vi "WRITE XNET Init Settings.vi"(7 "Unit Type":T1, 8 "error in (no error)":errorcluster, 9 "Box IDs":u8[](array[numeric])=[1], 10 "CAN Interface":refnum<k21>, 11 "XNET_BS120x in":refnum<class "XNET_BS120x.lvclass">) -> (0 "error out":errorcluster, 3 "XNET_BS120x out":refnum<class "XNET_BS120x.lvclass">)   [LabVIEW 2021, in "BS120x Driver.lvlib" / "XNET_BS120x.lvclass"]
uses:
  XNET_BS120x.lvclass
  XNET_BS120x.lvclass/XNET_BS120x.ctl
  TypeDefs/UnitType.ctl
  BS120x.lvclass
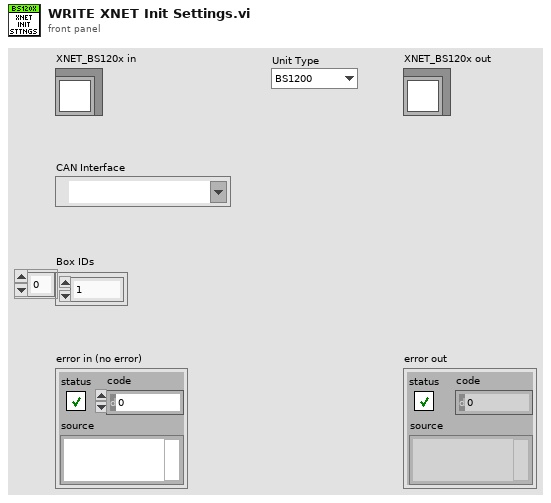
[diagram p1: front panel]
types:
  T1 = typedef "BS120x Driver.lvlib/BS120x.lvclass/UnitType.ctl" = enum16{"BS1200", "BS1201"}
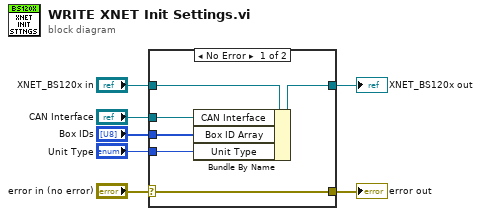
[diagram p0: block diagram]
diagram:
  n1 = case shown="No Error" "error in (no error)" {
    selector: "error in (no error)" -> [w12 w15]
    tunnel: [w12 w15] -> w6
    tunnel: [w11 w14] -> w4
    tunnel: "XNET_BS120x in" -> [w13 w14]
    tunnel: "CAN Interface" -> [w10 _]
    tunnel: "Box IDs" -> [w9 _]
    tunnel: "Unit Type" -> [w8 _]
    frame No Error {
      n2 = Bundle By Name(cluster=w13, "CAN Interface"=w10, "Box ID Array"=w9, "Unit Type"=w8) -> (w11:refnum<class "XNET_BS120x.lvclass">)
    }
    frame Error {
    }
  }
  "error out" <- w6
  "XNET_BS120x out" <- w4
